vi "DH Transformation.vi"(3 "n+1":T1 {"alpha (degrees)" format="%.2f"; "a" format="%.2f"; "d" format="%.2f"; "Theta (degrees)" format="%.2f"}) -> (1 "An+1":T2={"nx"=1.0, "ny"=0.0, "nz"=0.0, "nw"=0.0, "ox"=0.0, "oy"=1.0, "oz"=0.0, "ow"=0.0, "ax"=0.0, "ay"=0.0, "az"=1.0, "aw"=0.0, "Px"=0.0, "Py"=0.0, "Pz"=0.0, "Pw"=1.0} {"Pw" format="%.2f"; "Pz" format="%.2f"; "Py" format="%.2f"; "Px" format="%.2f"; "aw" format="%.2f"; "az" format="%.2f"; "ay" format="%.2f"; "ax" format="%.2f"; "ow" format="%.2f"; "nw" format="%.2f"; "oz" format="%.2f"; "oy" format="%.2f"; "ox" format="%.2f"; "nz" format="%.2f"; "ny" format="%.2f"; "nx" format="%.2f"})   [LabVIEW 2012]
uses:
  <userlib>/rosforlv/Gazebo/AxesDrawing/ReferenceFrame.ctl
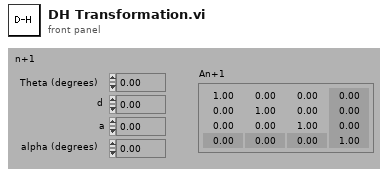
[diagram p1: front panel]
types:
  T1 = cluster{"Theta (degrees)":dbl, "d":dbl, "a":dbl, "alpha (degrees)":dbl}
  T2 = typedef "ReferenceFrame.ctl" = cluster{"nx":dbl, "ny":dbl, "nz":dbl, "nw":dbl, "ox":dbl, "oy":dbl, "oz":dbl, "ow":dbl, "ax":dbl, "ay":dbl, "az":dbl, "aw":dbl, "Px":dbl, "Py":dbl, "Pz":dbl, "Pw":dbl}
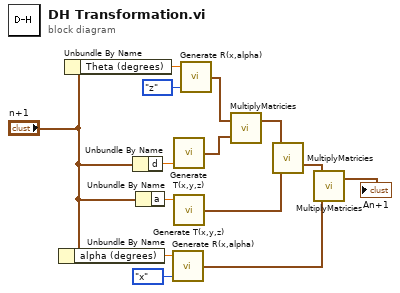
[diagram p0: block diagram]
diagram:
  n1 = Unbundle By Name("n+1") -> ("alpha (degrees)"=w3:dbl)
  n2 = Unbundle By Name("n+1") -> ("Theta (degrees)"=w13:dbl)
  n3 = Unbundle By Name("n+1") -> ("d"=w2:dbl)
  n4 = Unbundle By Name("n+1") -> ("a"=w1:dbl)
  n5 = call <userlib>:"Generate R(x,alpha).vi"("Axis"=enum16{"x", "y", "z"}."x", "Angle (degrees)"=w3) -> ("Final Frame"=w5:T2)  [unwired: 1 in]
  n6 = call <userlib>:"Generate T(x,y,z).vi"("Z"=w2) -> ("Final Frame"=w11:T2)  [unwired: 2 in]
  n7 = call <userlib>:"Generate T(x,y,z).vi"("X"=w1) -> ("Final Frame"=w8:T2)  [unwired: 2 in]
  n8 = call <userlib>:"Generate R(x,alpha).vi"("Axis"=enum16{"x", "y", "z"}."z", "Angle (degrees)"=w13) -> ("Final Frame"=w12:T2)  [unwired: 1 in]
  n9 = call <userlib>:"MultiplyMatricies.vi"("B"=w11, "A"=w12) -> ("AxB"=w9:T2)  [unwired: 1 out]
  n10 = call <userlib>:"MultiplyMatricies.vi"("B"=w8, "A"=w9) -> ("AxB"=w7:T2)  [unwired: 1 out]
  n11 = call <userlib>:"MultiplyMatricies.vi"("B"=w5, "A"=w7) -> ("AxB"=→"An+1":T2)  [unwired: 1 out]
